vi "JSON Top Level Search.vi"() -> ()   [LabVIEW 2013, in "LV JSON.lvlib"]
uses:
  LV JSON.lvlib
panel:
  out "concatenated string":string
  in  "Element to search for":string
  in  "String":string
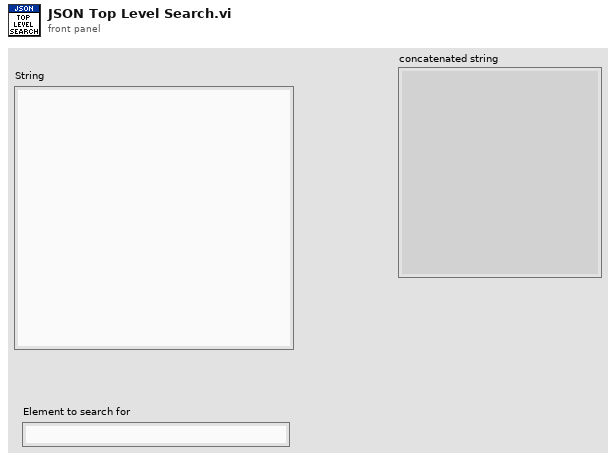
[diagram p1: front panel]
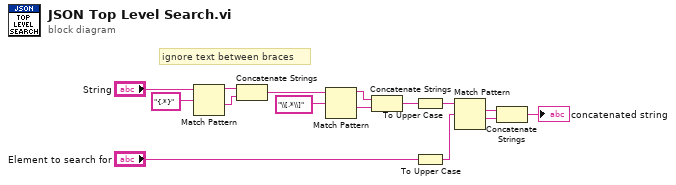
[diagram p0: block diagram]
diagram:
  # "ignore text between braces"
  n1 = Match Pattern(string="String", regular expression="{.*}") -> (before substring=w13:string, after substring=w12:string)  [unwired: 1 in, 2 out]
  n2 = Concatenate Strings(w13, w12) -> (w2:string)
  n3 = Match Pattern(string=w2, regular expression="\\[.*\\]") -> (before substring=w4:string, after substring=w5:string)  [unwired: 1 in, 2 out]
  n4 = Concatenate Strings(w4, w5) -> (w1:string)
  n5 = To Upper Case(1:w1) -> (0:w11:string)
  n6 = To Upper Case(1:"Element to search for") -> (0:w9:string)
  n7 = Match Pattern(string=w11, regular expression=w9) -> (match substring=w8:string, after substring=w7:string)  [unwired: 1 in, 2 out]
  n8 = Concatenate Strings(w8, w7) -> (→"concatenated string":string)
